vi "Save_Database.vi"(8 "error in":errorcluster, 11 "Database":T1[](array[typedef])) -> (0 "error out":errorcluster)   [LabVIEW 2022 SP3]
uses:
  Database_element.ctl
  <vilib>/Utility/file.llb/Write Delimited Spreadsheet (string).vi
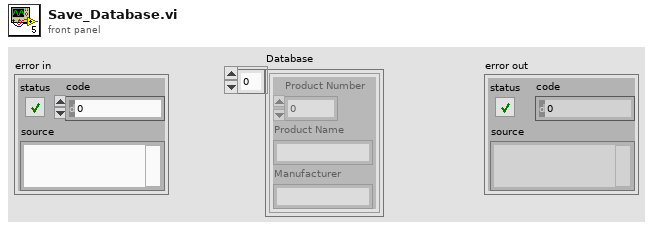
[diagram p1: front panel]
types:
  T1 = typedef "Database_element.ctl" = cluster{"Product Number":i32, "Product Name":string, "Manufacturer":string}
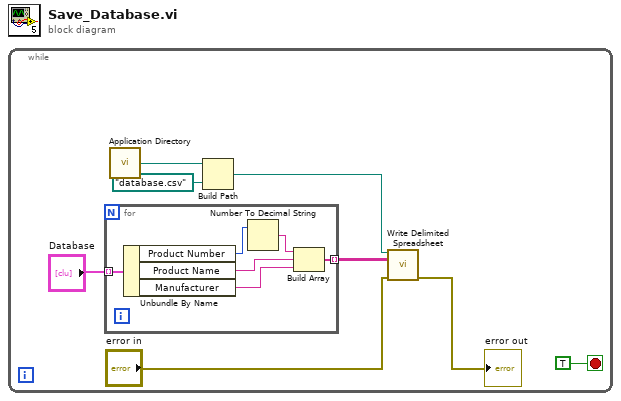
[diagram p0: block diagram]
diagram:
  n1 = while {
    stop <- TRUE stop-if-true
    n2 = for {
      tunnel: "Database" -> [w14] mode=indexing
      tunnel: [w11] -> w4 mode=indexing
      n3 = Unbundle By Name(w14) -> ("Product Number"=w10:i32, "Product Name"=w13:string, "Manufacturer"=w12:string)
      n4 = Number To Decimal String(number=w10) -> (decimal integer string=w9:string)  [unwired: 1 in]
      n5 = Build Array(w9, w13, w12) -> (w11:string[])
    }
    n6 = call <vilib>:"Application Directory.vi"() -> ("Application Directory"=w7:path)
    n7 = Build Path(base path=w7, name or relative path=path "database.csv") -> (appended path=w3:path)
    n8 = call-poly <vilib>:"Write Delimited Spreadsheet.vi"("file path (dialog if empty)"=w3, "2D data"=w4, "error in (no error)"="error in") -> ("error out"=→"error out":errorcluster)  [unwired: 11 in, 1 out]
  }
